vi "dfd_Convert Wordlength to Representation.vi"(4 "wl":i16) -> (1 "representation":T1(ring))   [LabVIEW 2017, in "NI_DigFilterLicensed.lvlib"]
uses:
  <vilib>/addons/Digital Filter Design/NI_DigFilterLicensed.lvlib
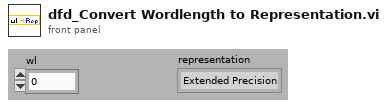
[diagram p1: front panel]
types:
  T1 = enum32{"Extended Precision", "Double Precision", "Single Precision", "Long", "Word", "Byte", "Unsigned Long", "Unsigned Word", "Unsigned Byte", "Complex Extended", "Complex Double", "Complex Single", "Quad", "Unsigned Quad"}
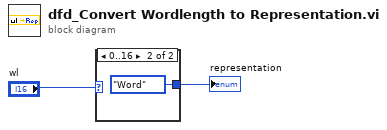
[diagram p0: block diagram]
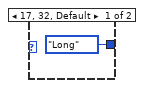
[diagram p2: hidden frame]
diagram:
  n1 = case shown="0..16" "wl" {
    tunnel: [T1."Long" ("new representation") T1."Word" ("new representation")] -> w2
    frame 17, 32, Default {
    }
    frame 0..16 {
    }
  }
  "representation" <- w2
